vi "手动界面.vi"(8 "错误输入（无错误）":errorcluster, 10 "界面切换队列":refnum<queue>, 11 "VISA资源名称输入":refnum<visa-resource-name>) -> (0 "错误输出":errorcluster, 3 "VISA资源名称输出":refnum<visa-resource-name>)   [LabVIEW 2018]
panel:
  out "毫秒计时值":u32
  in  "枚举":T1(ring)
  out "选项卡控件":enum32{"选项卡 1", "选项卡 2"}(tab)
  out "写R2E+读Y1C+2号吸嘴真空":bool
  out "写R2C+读Y1B+1号吸嘴真空":bool
  out "写R2A+读Y13+真空泵":bool
  out "写R81+读R81+切换+快速":bool
  out "写R2D+读Y16+2号吸嘴吹气":bool
  out "写R2B+读Y14+1号吸嘴吹气":bool
  out "烧录座手动界面":bool
  out "写R1F+读R5F+R2轴旋转定位":bool
  out "写R1C+读R5C+R1轴旋转定位":bool
  in  "DT63+枚举":enum16{"90度", "180度", "270度"}(ring)
  in  "DT62+枚举":enum16{"90度", "180度", "270度"}(ring)
  out "写R25+读YC+卷带信号":bool
  out "写R26+读YD+换盘信号":bool
  out "写R19+读R59+Z2轴+":bool
  out "写R16+读R56+Z轴+":bool
  out "写R168+读R168+切换+手柄Z1轴":bool
  out "写R1A+读R5A+Z2轴-":bool
  out "写R17+读R57+Z1轴-":bool
  out "写R20+读Y19+2#飞达信号":bool
  out "写R2F+读Y18+1#飞达信号":bool
  out "写R1B+读R5B+Z2轴回原点":bool
  out "写R18+读R58+Z轴回原点":bool
  out "手动2界面":bool
  out "写R80+读R80+报警清除":bool
  out "写R8+读R9+机器复位":bool
  out "写R4+读R4+手动停止":bool
  out "写R0+读R1+手动启动":bool
  out "写R11+读R51+X轴-":bool
  out "写R10+读R50+X轴+":bool
  out "写R13+读R53+Y轴+":bool
  out "写R14+读R54+Y轴-":bool
  out "写R15+读R55+Y轴回原点":bool
  out "写R12+读R52+X轴回原点":bool
  out "DDT90356":dbl
  out "DDT90348":dbl
  out "自动界面":bool
  out "手动界面":bool
  out "参数界面":bool
  out "IO界面":bool
  out "产品界面":bool
  out "字符串":string
  out "DDT90352":dbl
  out "DDT90360":dbl
  out "DT1184":T2(ring)
  out "通讯周期":dbl
  # "X"
  # "Z1"
  # "Z2"
  # "Y"
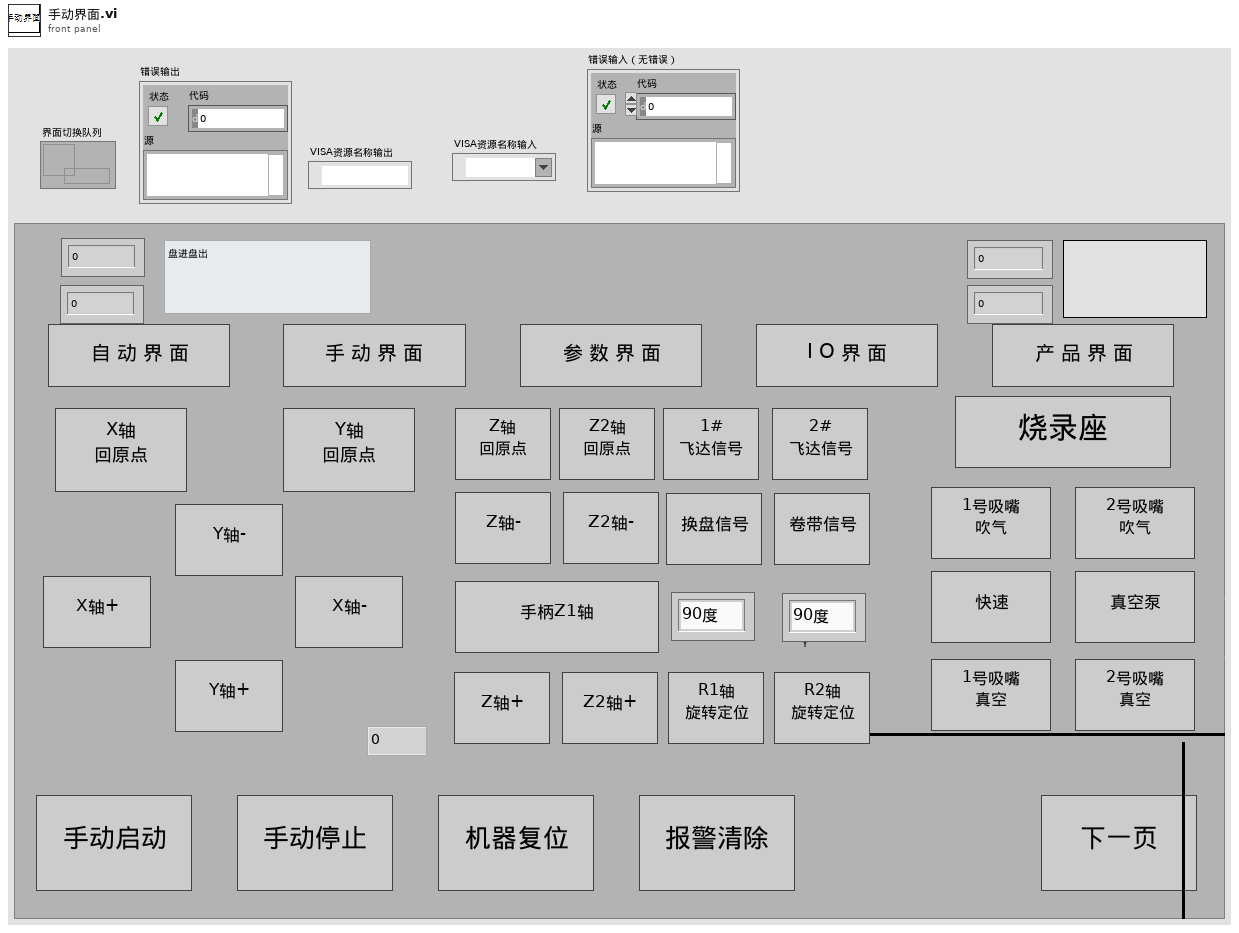
[diagram p1: front panel]
types:
  T1 = enum16{"读初始化", "读DT62+8", "读R168+8", "读R80+8", "读YC+8", "读Y1B+8", "读Y13+8", "读R9+8", "读R1+8", "读R50+8", "读R58+8", "读DDT90356", "读DT1184", "读DDT90348", ""}
  T2 = enum16{"盘进盘出", "卷进卷出", "盘进卷出", "管进盘出", "管进卷出", "卷进盘出", ""}
  T3 = enum8{"Enabled", "Disabled", "Disabled and Grayed Out"}
  T4 = typedef "数据簇.ctl" = cluster{"字符串":string, "数值":i32, "布尔":bool}
  T5 = typedef "lveventtype.ctl" = enum32{"Null", "Timeout", "Annotation Menu Selection", "Annotation Menu Selection?", "App Instance Close", "App Instance Close?", "Autoscale Range Change", "Bookmark Info Change", "Cell Edit", "Cell Edit?", "Cursor Grab", "Cursor Grab?", "Cursor Menu Selection", "Cursor Menu Selection?", "Cursor Move", "Cursor Release", "Data Change", "Direction Change", "Display State Change", "Drag Ended", "Drag Enter", "Drag Leave", "Drag Over", "Drag Source Update", "Drag Starting", "Drag Starting?", "Drop", "Exec State Change", "Key Down", "Key Down?", "Key Repeat", "Key Repeat?", "Key Up", "Listbox Double Click", "Menu Activation?", "Menu Selection (App)", "Menu Selection? (App)", "Menu Selection (User)", "Mouse Down", "Mouse Down?", "Mouse Enter", "Mouse Leave", "Mouse Move", "Mouse Up", "Mouse Wheel", "NI Security User Change (App)", "Pane Size", "Panel Close", "Panel Close?", "Panel Resize", "Plot Attribute Change", "Scale Range Change", "Shortcut Menu Activation?", "Shortcut Menu Selection (App)", "Shortcut Menu Selection? (App)", "Shortcut Menu Selection (User)", "Tree Double Click", "Tree Drag", "Tree Drag?", "Tree Drop", "Tree Drop?", "Tree Item Close", "Tree Item Close?", "Tree Item Open", "Tree Item Open?", "User Event", "Value Change"}
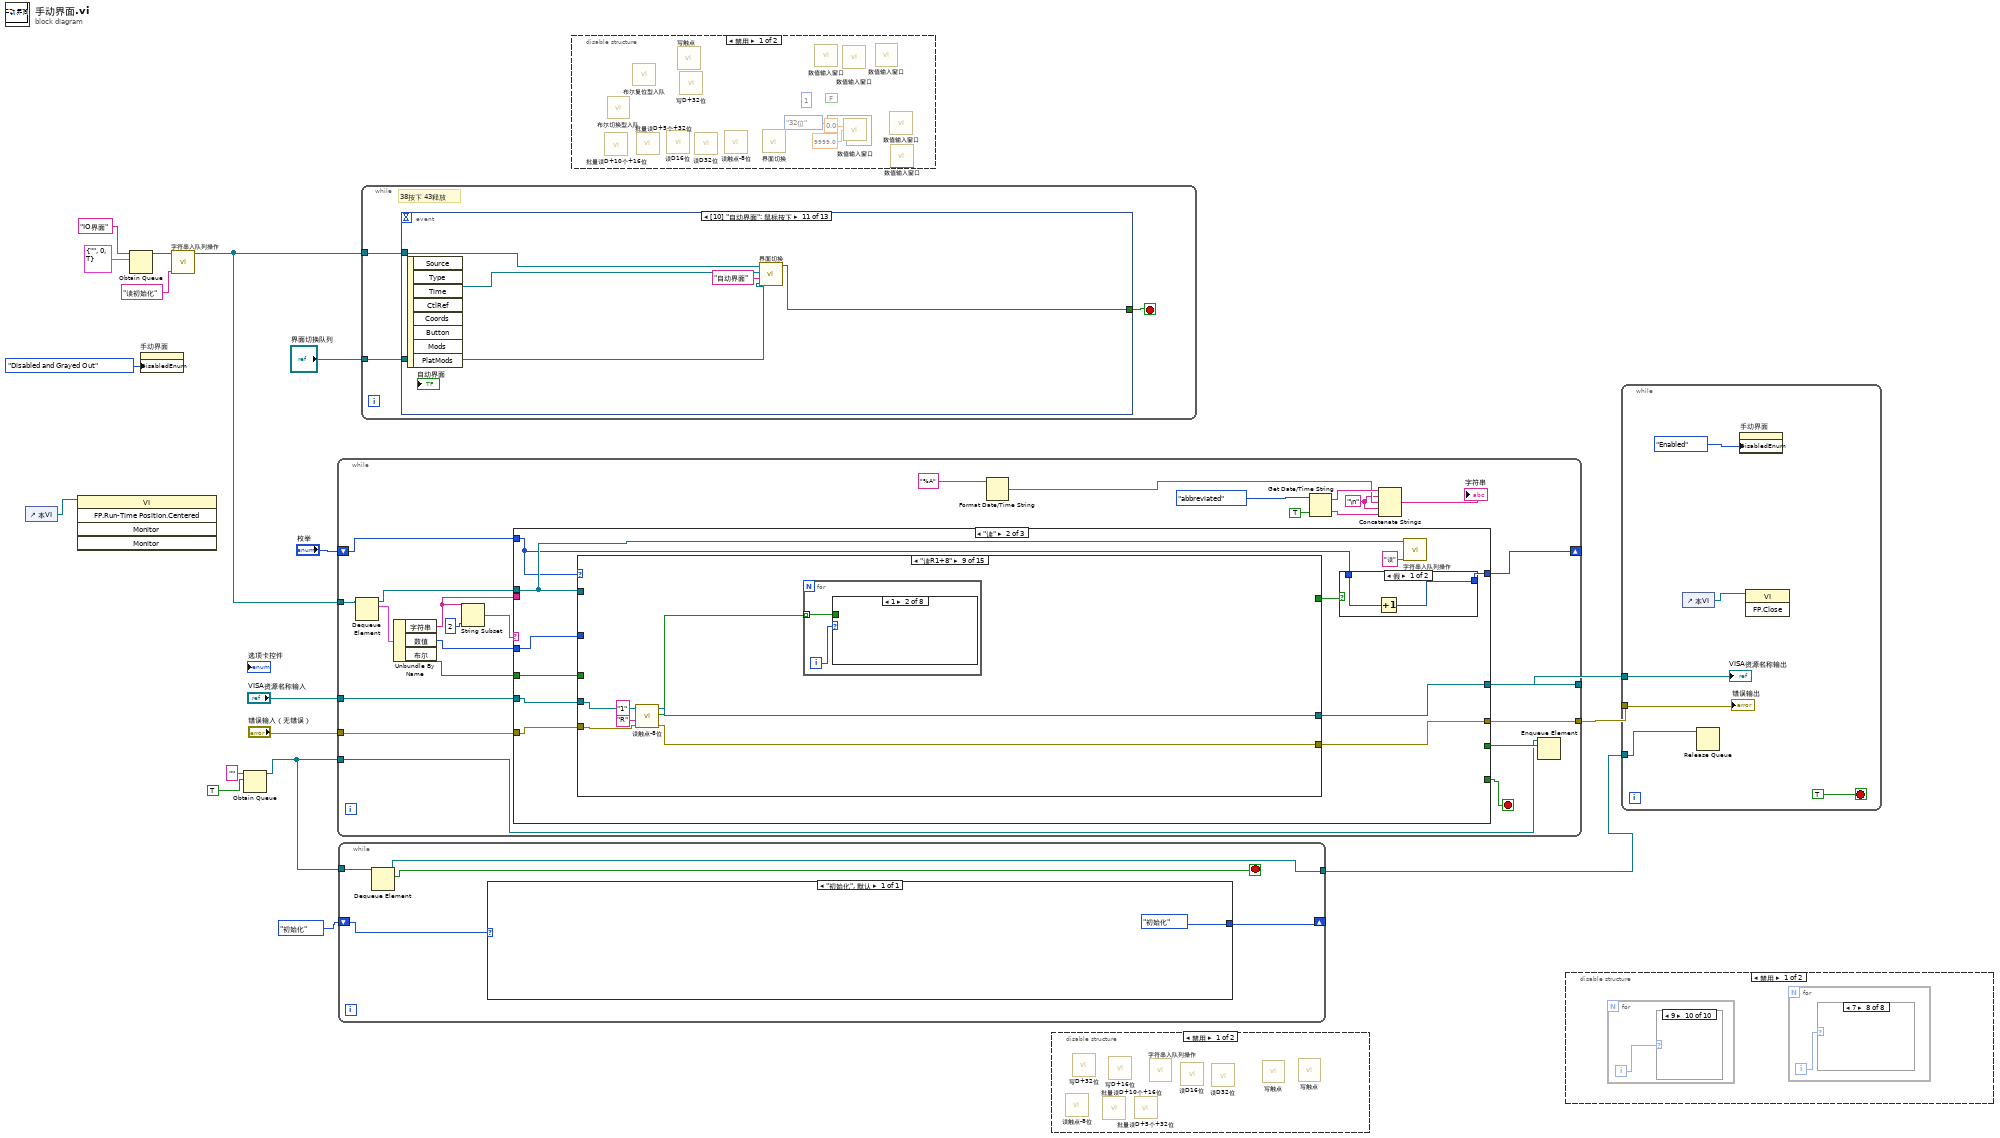
[diagram p0: block diagram]
diagram:
  n1 = control-ref of="本VI"() -> (w2:refnum<vi>)
  n2 = invoke class="VI" method="FP.Run-Time Position.Centered"(reference=w2) -> ()  [unwired: 4 in, 5 out]
  n3 = Obtain Queue(name (unnamed)="IO界面" ("名称（未命名）"), element data type=T4 {"字符串"="", "数值"=0, "布尔"=TRUE}) -> (queue out=w11:refnum<queue>)  [unwired: 3 in, 2 out]
  n4 = property on="手动界面" class="Bool"("DisabledEnum"=T3."Disabled and Grayed Out" ("禁用")) -> ()  [unwired: 2 in, 2 out]
  n5 = call "字符串入队列操作.vi"("字符消息入队列"="读初始化", "界面切换队列"=w11) -> ("队列输出"=w3:refnum<queue>)  [unwired: 9 in]
  n6 = Obtain Queue(name (unnamed)="" ("名称（未命名）"), element data type=TRUE) -> (queue out=w6:refnum<queue>)  [unwired: 3 in, 2 out]
  n7 = while {
    tunnel: w3 -> [w39]
    tunnel: "VISA资源名称输入" -> [w32]
    tunnel: "错误输入（无错误）" -> [w31]
    tunnel: [w30] -> w13
    tunnel: [w29] -> w12
    shift-right: [w26] -> _
    shift-left: "枚举" -> [w27]
    tunnel: w6 -> [w19]
    stop <- w21 stop-if-true
    w23 = "\n"
    n8 = Dequeue Element(queue=w39) -> (queue out=w36:refnum<queue>, element=w38:T4)  [unwired: 2 in, 2 out]
    n9 = Unbundle By Name(w38) -> ("字符串"=w33:string, "数值"=w35:i32, "布尔"=w34:bool)
    n10 = String Subset(string=w33, length (rest)=2 ("长度（剩余）")) -> (substring=w37:string)  [unwired: 1 in]
    n11 = case shown="\"读\"" w37 {
      selector: w37 -> [w46 _ _]
      tunnel: w36 -> [_ w54 w243]
      tunnel: w35 -> [_ w61 w242]
      tunnel: w34 -> [_ w60 w241]
      tunnel: w33 -> [_ _ w235]
      tunnel: w32 -> [w45 w59 w240]
      tunnel: w31 -> [w44 w58 w239]
      tunnel: [w45 w57 w237] -> w30
      tunnel: [w44 w56 w236] -> w29
      tunnel: [_ _ w238] -> w21
      tunnel: w27 -> [_ w52 _]
      tunnel: [_ w51 _] -> w26
      tunnel: [_ _ w233] -> w20
      frame "", Default {
        n12 = Concatenate Strings("无对应消息分支**" ("消息"), w46, "**" ("字符串"), "读写状态机" ("字符串")) -> (w48:string)
        n13 = One Button Dialog(message=w48) -> ()  [unwired: 1 in, 1 out]
      }
      frame "读" {
        n14 = case shown="\"读R1+8\"" w52 {
          tunnel: w54 -> [_ _ _ _ _ _ _ _ _ _ _ _ _ _ _]
          tunnel: w61 -> [_ _ _ _ _ _ _ _ _ _ _ _ _ _ _]
          tunnel: w59 -> [w66 w72 w83 w93 w104 w115 w126 w140 w150 w161 w178 w198 w207 w220 w232]
          tunnel: w58 -> [w65 w71 w82 w92 w103 w114 w125 w139 w149 w160 w177 w197 w206 w219 w231]
          tunnel: [w66 w69 w79 w91 w100 w113 w124 w136 w146 w157 w176 w196 w205 w218 w232] -> w57
          tunnel: [w65 w68 w78 w90 w99 w112 w123 w135 w145 w156 w175 w195 w204 w217 w231] -> w56
          tunnel: w60 -> [_ _ _ _ _ _ _ _ _ _ _ _ _ _ _]
          tunnel: [_ _ _ _ _ _ _ _ _ _ _ _ _ _ TRUE] -> w53
          frame "读初始化" {
            n15 = Tick Count (ms)() -> (millisecond timer value=→"毫秒计时值":u32)
          }
          frame "读DT62+8" {
            n16 = call "批量读D+10个+16位.vi"("error out"=w71, "读取D地址"=62, "VISA resource name out"=w72) -> ("error IO"=w68:errorcluster, "数组"=w67:i32[], "VISA resource name out 2"=w69:refnum<visa-resource-name>)  [unwired: 5 in, 1 out]
            n17 = for {
              tunnel: w67 -> [w73] mode=indexing
              i -> [w74]
              n18 = case shown="1" w74 {
                tunnel: w73 -> [w75 w76 _ _ _ _ _ _ _ _]
                frame 0, Default {
                  n19 = local write "DT62+枚举"(w75) -> ()
                }
                frame 1 {
                  n20 = local write "DT63+枚举"(w76) -> ()
                }
                frame 2 {
                }
                frame 3 {
                }
                frame 4 {
                }
                frame 5 {
                }
                frame 6 {
                }
                frame 7 {
                }
                frame 8 {
                }
                frame 9 {
                }
              }
            }
          }
          frame "读R168+8" {
            n21 = call "读触点-8位.vi"("error out"=w82, "触点类型"="R", "读取起始地址"="168", "VISA resource name out"=w83) -> ("error IO"=w78:errorcluster, "读取布尔数组"=w77:bool[], "VISA resource name out 2"=w79:refnum<visa-resource-name>)  [unwired: 4 in, 1 out]
            n22 = for {
              tunnel: w77 -> [w84] mode=indexing
              i -> [w85]
              n23 = case shown="0, 默认" w85 {
                tunnel: w84 -> [w86 _ _ _ _ _ _ _]
                frame 0, Default {
                  "写R168+读R168+切换+手柄Z1轴" <- w86
                }
                frame 1 {
                }
                frame 2 {
                }
                frame 3 {
                }
                frame 4 {
                }
                frame 5 {
                }
                frame 6 {
                }
                frame 7 {
                }
              }
            }
          }
          frame "读R80+8" {
            n24 = call "读触点-8位.vi"("error out"=w92, "触点类型"="R", "读取起始地址"="80", "VISA resource name out"=w93) -> ("error IO"=w90:errorcluster, "读取布尔数组"=w87:bool[], "VISA resource name out 2"=w91:refnum<visa-resource-name>)  [unwired: 4 in, 1 out]
            n25 = for {
              tunnel: w87 -> [w94] mode=indexing
              i -> [w95]
              n26 = case shown="0, 默认" w95 {
                tunnel: w94 -> [w96 w97 _ _ _ _ _ _]
                frame 0, Default {
                  "写R80+读R80+报警清除" <- w96
                }
                frame 1 {
                  "写R81+读R81+切换+快速" <- w97
                }
                frame 2 {
                }
                frame 3 {
                }
                frame 4 {
                }
                frame 5 {
                }
                frame 6 {
                }
                frame 7 {
                }
              }
            }
          }
          frame "读YC+8" {
            n27 = call "读触点-8位.vi"("error out"=w103, "触点类型"="Y", "读取起始地址"="C", "VISA resource name out"=w104) -> ("error IO"=w99:errorcluster, "读取布尔数组"=w98:bool[], "VISA resource name out 2"=w100:refnum<visa-resource-name>)  [unwired: 4 in, 1 out]
            n28 = for {
              tunnel: w98 -> [w105] mode=indexing
              i -> [w106]
              n29 = case shown="1" w106 {
                tunnel: w105 -> [w107 w108 _ _ _ _ _ _]
                frame 0, Default {
                  "写R25+读YC+卷带信号" <- w107
                }
                frame 1 {
                  "写R26+读YD+换盘信号" <- w108
                }
                frame 2 {
                }
                frame 3 {
                }
                frame 4 {
                }
                frame 5 {
                }
                frame 6 {
                }
                frame 7 {
                }
              }
            }
          }
          frame "读Y1B+8" {
            n30 = call "读触点-8位.vi"("error out"=w114, "触点类型"="Y", "读取起始地址"="1C", "VISA resource name out"=w115) -> ("error IO"=w112:errorcluster, "读取布尔数组"=w111:bool[], "VISA resource name out 2"=w113:refnum<visa-resource-name>)  [unwired: 4 in, 1 out]
            n31 = for {
              tunnel: w111 -> [w116] mode=indexing
              i -> [w117]
              n32 = case shown="1" w117 {
                tunnel: w116 -> [w118 w119 _ _ _ _ _ _]
                frame 0, Default {
                  "写R2C+读Y1B+1号吸嘴真空" <- w118
                }
                frame 1 {
                  "写R2E+读Y1C+2号吸嘴真空" <- w119
                }
                frame 2 {
                }
                frame 3 {
                }
                frame 4 {
                }
                frame 5 {
                }
                frame 6 {
                }
                frame 7 {
                }
              }
            }
          }
          frame "读Y13+8" {
            n33 = call "读触点-8位.vi"("error out"=w125, "触点类型"="Y", "读取起始地址"="13", "VISA resource name out"=w126) -> ("error IO"=w123:errorcluster, "读取布尔数组"=w122:bool[], "VISA resource name out 2"=w124:refnum<visa-resource-name>)  [unwired: 4 in, 1 out]
            n34 = for {
              tunnel: w122 -> [w127] mode=indexing
              i -> [w128]
              n35 = case shown="6" w128 {
                tunnel: w127 -> [w129 w130 _ w131 _ w132 w133 _]
                frame 0, Default {
                  "写R2A+读Y13+真空泵" <- w129
                }
                frame 1 {
                  "写R2B+读Y14+1号吸嘴吹气" <- w130
                }
                frame 2 {
                }
                frame 3 {
                  "写R2D+读Y16+2号吸嘴吹气" <- w131
                }
                frame 4 {
                }
                frame 5 {
                  "写R2F+读Y18+1#飞达信号" <- w132
                }
                frame 6 {
                  "写R20+读Y19+2#飞达信号" <- w133
                }
                frame 7 {
                }
              }
            }
          }
          frame "读R9+8" {
            n36 = call "读触点-8位.vi"("error out"=w139, "触点类型"="R", "读取起始地址"="9", "VISA resource name out"=w140) -> ("error IO"=w135:errorcluster, "读取布尔数组"=w134:bool[], "VISA resource name out 2"=w136:refnum<visa-resource-name>)  [unwired: 4 in, 1 out]
            n37 = for {
              tunnel: w134 -> [w141] mode=indexing
              i -> [w142]
              n38 = case shown="0, 默认" w142 {
                tunnel: w141 -> [w143 _ _ _ _ _ _ _]
                frame 0, Default {
                  "写R8+读R9+机器复位" <- w143
                }
                frame 1 {
                }
                frame 2 {
                }
                frame 3 {
                }
                frame 4 {
                }
                frame 5 {
                }
                frame 6 {
                }
                frame 7 {
                }
              }
            }
          }
          frame "读R1+8" {
            n39 = call "读触点-8位.vi"("error out"=w149, "触点类型"="R", "读取起始地址"="1", "VISA resource name out"=w150) -> ("error IO"=w145:errorcluster, "读取布尔数组"=w144:bool[], "VISA resource name out 2"=w146:refnum<visa-resource-name>)  [unwired: 4 in, 1 out]
            n40 = for {
              tunnel: w144 -> [w151] mode=indexing
              i -> [w152]
              n41 = case shown="1" w152 {
                tunnel: w151 -> [w153 _ _ w154 _ _ _ _]
                frame 0, Default {
                  "写R0+读R1+手动启动" <- w153
                }
                frame 1 {
                }
                frame 2 {
                }
                frame 3 {
                  "写R4+读R4+手动停止" <- w154
                }
                frame 4 {
                }
                frame 5 {
                }
                frame 6 {
                }
                frame 7 {
                }
              }
            }
          }
          frame "读R50+8" {
            n42 = call "读触点-8位.vi"("error out"=w160, "触点类型"="R", "读取起始地址"="50", "VISA resource name out"=w161) -> ("error IO"=w156:errorcluster, "读取布尔数组"=w155:bool[], "VISA resource name out 2"=w157:refnum<visa-resource-name>)  [unwired: 4 in, 1 out]
            n43 = for {
              tunnel: w155 -> [w162] mode=indexing
              i -> [w163]
              n44 = case shown="7" w163 {
                tunnel: w162 -> [w164 w165 w166 w167 w168 w169 w170 w171]
                frame 0, Default {
                  "写R10+读R50+X轴+" <- w164
                }
                frame 1 {
                  "写R11+读R51+X轴-" <- w165
                }
                frame 2 {
                  "写R12+读R52+X轴回原点" <- w166
                }
                frame 3 {
                  "写R13+读R53+Y轴+" <- w167
                }
                frame 4 {
                  "写R14+读R54+Y轴-" <- w168
                }
                frame 5 {
                  "写R15+读R55+Y轴回原点" <- w169
                }
                frame 6 {
                  "写R16+读R56+Z轴+" <- w170
                }
                frame 7 {
                  "写R17+读R57+Z1轴-" <- w171
                }
              }
            }
          }
          frame "读R58+8" {
            n45 = call "读触点-8位.vi"("error out"=w177, "触点类型"="R", "读取起始地址"="58", "VISA resource name out"=w178) -> ("error IO"=w175:errorcluster, "读取布尔数组"=w172:bool[], "VISA resource name out 2"=w176:refnum<visa-resource-name>)  [unwired: 4 in, 1 out]
            n46 = for {
              tunnel: w172 -> [w179] mode=indexing
              i -> [w180]
              n47 = case shown="7" w180 {
                tunnel: w179 -> [w181 w182 w183 w184 w185 _ _ w186]
                frame 0, Default {
                  "写R18+读R58+Z轴回原点" <- w181
                }
                frame 1 {
                  "写R19+读R59+Z2轴+" <- w182
                }
                frame 2 {
                  "写R1A+读R5A+Z2轴-" <- w183
                }
                frame 3 {
                  "写R1B+读R5B+Z2轴回原点" <- w184
                }
                frame 4 {
                  "写R1C+读R5C+R1轴旋转定位" <- w185
                }
                frame 5 {
                }
                frame 6 {
                }
                frame 7 {
                  "写R1F+读R5F+R2轴旋转定位" <- w186
                }
              }
            }
          }
          frame "读DDT90356" {
            n48 = call "批量读D+5个+32位.vi"("error out"=w197, "读取D地址"=90356, "VISA resource name out"=w198) -> ("error IO"=w195:errorcluster, "数组"=w201:i32[], "VISA resource name out 2"=w196:refnum<visa-resource-name>)  [unwired: 5 in, 1 out]
            n49 = Index Array(array=w201, index #1=0 ("索引"), index #2=2 ("索引")) -> (element #1=w194:i32, element #2=w193:i32)
            n50 = To Double Precision Float(number=w194) -> (double precision float=w192:dbl)
            n51 = To Double Precision Float(number=w193) -> (double precision float=w189:dbl)
            n52 = Divide(x=w192, y=100.0) -> (x/y=→"DDT90356":dbl)
            n53 = Divide(x=w189, y=100.0) -> (x/y=→"DDT90360":dbl)
          }
          frame "读DT1184" {
            n54 = call "读D16位.vi"("error out"=w206, "读取D地址"=1184, "VISA resource name out"=w207) -> ("error IO"=w204:errorcluster, "数值"=→"DT1184":u32, "VISA resource name out 2"=w205:refnum<visa-resource-name>)  [unwired: 5 in, 1 out]
          }
          frame "读DDT90348" {
            n55 = call "批量读D+5个+32位.vi"("error out"=w219, "读取D地址"=90348, "VISA resource name out"=w220) -> ("error IO"=w217:errorcluster, "数组"=w224:i32[], "VISA resource name out 2"=w218:refnum<visa-resource-name>)  [unwired: 5 in, 1 out]
            n56 = Index Array(array=w224, index #1=0 ("索引"), index #2=2 ("索引")) -> (element #1=w216:i32, element #2=w215:i32)
            n57 = To Double Precision Float(number=w215) -> (double precision float=w210:dbl)
            n58 = To Double Precision Float(number=w216) -> (double precision float=w214:dbl)
            n59 = Divide(x=w210, y=100.0) -> (x/y=→"DDT90352":dbl)
            n60 = Divide(x=w214, y=100.0) -> (x/y=→"DDT90348":dbl)
          }
          frame "" {
            n61 = local read "毫秒计时值"() -> (w228:u32)
            n62 = Tick Count (ms)() -> (millisecond timer value=w229:u32)
            n63 = Subtract(x=w229, y=w228) -> (x-y=w227:u32)
            n64 = Divide(x=w227, y=u32 1000) -> (x/y=→"通讯周期":dbl)
          }
        }
        n65 = case shown="假" w53 {
          tunnel: w52 -> [w63 _]
          tunnel: [w62 _] -> w51
          frame False {
            n66 = Increment(x=w63) -> (x+1=w62:T1)
          }
          frame True {
          }
        }
        n67 = call "字符串入队列操作.vi"("字符消息入队列"="读", "界面切换队列"=w54) -> ()  [unwired: 9 in, 1 out]
      }
      frame "写" {
        n68 = call "状态匹配.vi"("输入状态"=w235) -> ("输出状态"=w234:string)  [unwired: 10 in]
        n69 = case shown="\"写DT\"" w234 {
          selector: w234 -> [w246 _ _ _ _]
          tunnel: w243 -> [_ _ _ _ w286]
          tunnel: w242 -> [_ w252 w269 _ _]
          tunnel: w241 -> [_ _ _ w280 _]
          tunnel: w240 -> [w245 w262 w273 w285 w291]
          tunnel: w239 -> [w244 w261 w272 w284 w290]
          tunnel: [_ _ _ _ w289] -> w238
          tunnel: [w245 w260 w271 w283 w291] -> w237
          tunnel: [w244 w259 w270 w282 w290] -> w236
          tunnel: w235 -> [_ w251 w263 w274 _]
          tunnel: [_ _ _ _ w289] -> w233
          frame "", Default {
            n70 = Concatenate Strings("无对应消息分支**" ("消息"), w246, "**" ("字符串"), "写状态机" ("字符串")) -> (w250:string)
            n71 = One Button Dialog(message=w250) -> ()  [unwired: 1 in, 1 out]
          }
          frame "写DT" {
            n72 = String Length(string=w251) -> (length=w257:i32)
            n73 = Subtract(x=w257, y=4) -> (x-y=w255:i32)
            n74 = String Subset(string=w251, offset (0)=4 ("偏移量(0)"), length (rest)=w255) -> (substring=w254:string)
            n75 = Decimal String To Number(string=w254) -> (number=w253:i32)  [unwired: 2 in, 1 out]
            n76 = call "写D+16位.vi"("error out"=w261, "输入数值"=w252, "输入地址D"=w253, "VISA resource name out"=w262) -> ("error out 2"=w259:errorcluster, "VISA resource name out 2"=w260:refnum<visa-resource-name>)  [unwired: 3 in, 3 out]
          }
          frame "写DDT" {
            n77 = String Length(string=w263) -> (length=w267:i32)
            n78 = Subtract(x=w267, y=5) -> ()  [unwired: 1 out]
            n79 = String Subset(string=w263, offset (0)=5 ("偏移量(0)")) -> (substring=w264:string)  [unwired: 1 in]
            n80 = Decimal String To Number(string=w264) -> (number=w265:i32)  [unwired: 2 in, 1 out]
            n81 = call "写D+32位.vi"("error out"=w272, "输入数值"=w269, "输入地址D"=w265, "VISA resource name out"=w273) -> ("error out 2"=w270:errorcluster, "VISA resource name out 2"=w271:refnum<visa-resource-name>)  [unwired: 4 in, 2 out]
          }
          frame "写R" {
            n82 = String Length(string=w274) -> (length=w278:i32)
            n83 = Subtract(x=w278, y=3) -> (x-y=w276:i32)
            n84 = String Subset(string=w274, offset (0)=3 ("偏移量(0)"), length (rest)=w276) -> (substring=w275:string)
            n85 = call "写触点.vi"("布尔"=w280, "error out"=w284, "触点类型"="R", "写入起始地址"=w275, "VISA resource name out"=w285) -> ("error IO"=w282:errorcluster, "VISA resource name out 2"=w283:refnum<visa-resource-name>)  [unwired: 4 in, 1 out]
          }
          frame "写退出" {
            w289 = TRUE
            n86 = Flush Queue(queue=w286) -> (queue out=w287:refnum<queue>, error out=w288:errorcluster)  [unwired: 1 in, 1 out]
            n87 = Release Queue(queue=w287, error in (no error)=w288) -> ()  [unwired: 1 in, 3 out]
          }
        }
      }
    }
    n88 = Format Date/Time String(time format string (%c)="%A" ("时间格式字符串(%c)")) -> (date/time string=w24:string)  [unwired: 2 in]
    n89 = Get Date/Time String(date format (0)=enum16{"short", "long", "abbreviated"}."abbreviated" ("日期格式(0)"), want seconds? (F)=TRUE ("需要秒？(F)")) -> (date string=w41:string, time string=w22:string)  [unwired: 1 in]
    n90 = Concatenate Strings(w41, w23, w24, w23, w22) -> (→"字符串":string)
    n91 = Enqueue Element(queue=w19, element=w20) -> ()  [unwired: 2 in, 3 out]
  }
  n92 = while {
    shift-right: [w295] -> _
    shift-left: enum16{"初始化"}."初始化" -> [w296]
    tunnel: w6 -> [w294]
    tunnel: [w292] -> w5
    stop <- w293 stop-if-true
    n93 = Dequeue Element(queue=w294) -> (queue out=w292:refnum<queue>, element=w293:bool)  [unwired: 2 in, 2 out]
    n94 = case shown="\"初始化\", 默认" w296 {
      tunnel: [enum16{"初始化"}."初始化"] -> w295
      frame "初始化", Default {
      }
    }
  }
  n95 = while {
    tunnel: w3 -> [w299]
    tunnel: "界面切换队列" -> [w298]
    stop <- w300 stop-if-true
    # "38按下 43释放"
    n96 = event shown="[10] \"自动界面\": 鼠标按下" {
      selector: _ -> [_ _ _ _ _ _ _ _ _ _ _ _ _]
      dyn-events: _ -> [_ _ _ _ _ _ _ _ _ _ _ _ _]
      timeout: _ -> [_ _ _ _ _ _ _ _ _ _ _ _ _]
      tunnel: [w304 _ _ w316 _ _ w331 w340 w345 w346 w355 _ w358] -> w300
      tunnel: w299 -> [w305 w308 w315 w320 w327 w330 w335 w339 w344 w350 w354 _ w357]
      tunnel: w298 -> [w303 _ _ w319 _ _ w334 w338 w343 w349 w353 _ w356]
      event "IO界面": Mouse Down {
        n97 = event-data() -> ("CtlRef"=w302:refnum<vi>)  [unwired: 1 in, 7 out]
        n98 = call "界面切换.vi"("界面切换队列输入"=w303, "切换界面名称输入"="IO界面", "Bool引用句柄"=w302, "状态转移输入"=w305) -> ("布尔"=w304:bool)  [unwired: 7 in]
      }
      event "DT62+枚举": Value Change {
        n99 = event-data() -> ("NewVal"=w306:enum16{"90度", "180度", "270度"})  [unwired: 1 in, 5 out]
        n100 = call "字符串入队列操作.vi"("字符消息入队列"="写DT62", "数值"=w306, "界面切换队列"=w308) -> ()  [unwired: 8 in, 1 out]
      }
      event "写R12+读R52+X轴回原点", "写R15+读R55+Y轴回原点", "写R14+读R54+Y轴-", "写R13+读R53+Y轴+", "写R10+读R50+X轴+", "写R11+读R51+X轴-", "写R0+读R1+手动启动", "写R4+读R4+手动停止", "写R8+读R9+机器复位", "写R80+读R80+报警清除", "写R18+读R58+Z轴回原点", "写R1B+读R5B+Z2轴回原点", "写R2F+读Y18+1#飞达信号", "写R20+读Y19+2#飞达信号", "写R17+读R57+Z1轴-", "写R1A+读R5A+Z2轴-", "写R16+读R56+Z轴+", "写R19+读R59+Z2轴+", "写R26+读YD+换盘信号", "写R25+读YC+卷带信号", "写R1C+读R5C+R1轴旋转定位", "写R1F+读R5F+R2轴旋转定位", "写R2B+读Y14+1号吸嘴吹气", "写R2D+读Y16+2号吸嘴吹气", "写R2A+读Y13+真空泵", "写R2C+读Y1B+1号吸嘴真空", "写R2E+读Y1C+2号吸嘴真空": Mouse Down; "写R12+读R52+X轴回原点", "写R15+读R55+Y轴回原点", "写R14+读R54+Y轴-", "写R13+读R53+Y轴+", "写R10+读R50+X轴+", "写R11+读R51+X轴-", "写R0+读R1+手动启动", "写R8+读R9+机器复位", "写R80+读R80+报警清除", "写R18+读R58+Z轴回原点", "写R1B+读R5B+Z2轴回原点", "写R2F+读Y18+1#飞达信号", "写R20+读Y19+2#飞达信号", "写R17+读R57+Z1轴-", "写R1A+读R5A+Z2轴-", "写R16+读R56+Z轴+", "写R19+读R59+Z2轴+", "写R26+读YD+换盘信号", "写R25+读YC+卷带信号", "写R1C+读R5C+R1轴旋转定位", "写R2B+读Y14+1号吸嘴吹气", "写R2D+读Y16+2号吸嘴吹气", "写R2A+读Y13+真空泵", "写R2C+读Y1B+1号吸嘴真空", "写R2E+读Y1C+2号吸嘴真空", "写R4+读R4+手动停止": Mouse Up {
        n101 = event-data() -> ("Type"=w314:T5, "CtlRef"=w313:refnum<vi>)  [unwired: 1 in, 6 out]
        n102 = property class="Bool"(reference=w313) -> (reference out=w310:refnum<vi>, "Label.Text"=w312:string)  [unwired: 1 in, 1 out]
        n103 = Match Pattern(string=w312, regular expression="+" ("正则表达式")) -> (before substring=w309:string)  [unwired: 1 in, 3 out]
        n104 = call "布尔复位型入队.vi"("队列输入"=w315, "数值"=w314, "控件引用"=w310, "字符消息入队列"=w309) -> ()  [unwired: 2 in, 3 out]
      }
      event "烧录座手动界面": Mouse Down {
        n105 = event-data() -> ("CtlRef"=w318:refnum<vi>)  [unwired: 1 in, 7 out]
        n106 = call "界面切换.vi"("界面切换队列输入"=w319, "切换界面名称输入"="烧录座手动界面", "Bool引用句柄"=w318, "状态转移输入"=w320) -> ("布尔"=w316:bool)  [unwired: 7 in]
      }
      event "写R81+读R81+切换+快速", "写R168+读R168+切换+手柄Z1轴": Mouse Down {
        n107 = event-data() -> ("CtlRef"=w323:refnum<vi>)  [unwired: 1 in, 7 out]
        n108 = property class="Bool"(reference=w323) -> (reference out=w322:refnum<vi>, "Label.Text"=w325:string)  [unwired: 1 in, 1 out]
        n109 = Match Pattern(string=w325, regular expression="+" ("正则表达式")) -> (before substring=w321:string)  [unwired: 1 in, 3 out]
        n110 = call "布尔切换型入队.vi"("字符串"=w321, "true启用入队"=TRUE, "控件引用"=w322, "消息入队列"=w327) -> ()  [unwired: 8 in]
      }
      event "DT63+枚举": Value Change {
        n111 = event-data() -> ("NewVal"=w328:enum16{"90度", "180度", "270度"})  [unwired: 1 in, 5 out]
        n112 = call "字符串入队列操作.vi"("字符消息入队列"="写DT63", "数值"=w328, "界面切换队列"=w330) -> ()  [unwired: 8 in, 1 out]
      }
      event "手动2界面": Mouse Down {
        n113 = event-data() -> ("CtlRef"=w333:refnum<vi>)  [unwired: 1 in, 7 out]
        n114 = call "界面切换.vi"("界面切换队列输入"=w334, "切换界面名称输入"="手动2界面", "Bool引用句柄"=w333, "状态转移输入"=w335) -> ("布尔"=w331:bool)  [unwired: 7 in]
      }
      event "参数界面": Mouse Down {
        n115 = event-data() -> ("CtlRef"=w337:refnum<vi>)  [unwired: 1 in, 7 out]
        n116 = call "界面切换.vi"("界面切换队列输入"=w338, "切换界面名称输入"="参数界面", "Bool引用句柄"=w337, "状态转移输入"=w339) -> ("布尔"=w340:bool)  [unwired: 7 in]
      }
      event "产品界面": Mouse Down {
        n117 = event-data() -> ("CtlRef"=w342:refnum<vi>)  [unwired: 1 in, 7 out]
        n118 = call "界面切换.vi"("界面切换队列输入"=w343, "切换界面名称输入"="产品界面", "Bool引用句柄"=w342, "状态转移输入"=w344) -> ("布尔"=w345:bool)  [unwired: 7 in]
      }
      event "手动界面": Mouse Down {
        n119 = event-data() -> ("CtlRef"=w348:refnum<vi>)  [unwired: 1 in, 7 out]
        n120 = call "界面切换.vi"("界面切换队列输入"=w349, "切换界面名称输入"="手动界面", "Bool引用句柄"=w348, "状态转移输入"=w350) -> ("布尔"=w346:bool)  [unwired: 7 in]
      }
      event "自动界面": Mouse Down {
        n121 = event-data() -> ("CtlRef"=w352:refnum<vi>)  [unwired: 1 in, 7 out]
        n122 = call "界面切换.vi"("界面切换队列输入"=w353, "切换界面名称输入"="自动界面", "Bool引用句柄"=w352, "状态转移输入"=w354) -> ("布尔"=w355:bool)  [unwired: 7 in]
      }
      event Timeout {
        n123 = event-data() -> ()  [unwired: 1 in, 3 out]
      }
      event Panel Close? {
        n124 = event-data() -> ()  [unwired: 1 in, 4 out]
        n125 = Two Button Dialog(message="确定退出程序？" ("消息")) -> (T button?=w359:bool)  [unwired: 2 in]
        n126 = case shown="真" w359 {
          tunnel: [_ TRUE] -> w358
          tunnel: w357 -> [_ w364]
          tunnel: w356 -> [_ w363]
          frame False {
          }
          frame True {
            n127 = call "字符串入队列操作.vi"("字符消息入队列"="退出", "界面切换队列"=w363) -> ()  [unwired: 9 in, 1 out]
            n128 = call "字符串入队列操作.vi"("字符消息入队列"="写退出", "界面切换队列"=w364) -> ()  [unwired: 9 in, 1 out]
          }
        }
        n129 = event-data("Discard?"=TRUE ("放弃？")) -> ()  [unwired: 1 in, 1 out]
      }
    }
  }
  n130 = disable-structure shown="禁用" {
    frame Disabled {
      (unwired) u32 1 ("转换比例")
      (unwired) FALSE ("忽略数值上下限")
      n131 = call "批量读D+10个+16位.vi"() -> ()  [unwired: 8 in, 4 out]
      n132 = call "布尔切换型入队.vi"() -> ()  [unwired: 12 in]
      n133 = call "布尔复位型入队.vi"() -> ()  [unwired: 6 in, 3 out]
      n134 = call "批量读D+5个+32位.vi"() -> ()  [unwired: 8 in, 4 out]
      n135 = call "读D16位.vi"() -> ()  [unwired: 8 in, 4 out]
      n136 = call "写触点.vi"() -> ()  [unwired: 9 in, 3 out]
      n137 = call "写D+32位.vi"() -> ()  [unwired: 8 in, 4 out]
      n138 = call "读D32位.vi"() -> ()  [unwired: 9 in, 3 out]
      n139 = call "读触点-8位.vi"() -> ()  [unwired: 8 in, 4 out]
      n140 = call "界面切换.vi"() -> ()  [unwired: 11 in, 1 out]
      n141 = call "数值输入窗口.vi"() -> ()  [unwired: 13 in, 3 out]
      n142 = call "数值输入窗口.vi"() -> ()  [unwired: 13 in, 3 out]
      n143 = call "数值输入窗口.vi"("输入下限"=0.0, "输入上限"=9999.0, "数据类型"=enum16{"32位", "16位"}."32位") -> ("转换比例"=w370:u32)  [unwired: 9 in, 3 out]
      n144 = call "数值输入窗口.vi"() -> ()  [unwired: 13 in, 3 out]
      n145 = call "数值输入窗口.vi"() -> ()  [unwired: 13 in, 3 out]
      n146 = call "数值输入窗口.vi"() -> ()  [unwired: 13 in, 3 out]
    }
    frame Enabled {
    }
  }
  n147 = disable-structure shown="禁用" {
    frame Disabled {
      n148 = call "读触点-8位.vi"() -> ()  [unwired: 8 in, 4 out]
      n149 = call "写D+32位.vi"() -> ()  [unwired: 8 in, 4 out]
      n150 = call "批量读D+10个+16位.vi"() -> ()  [unwired: 8 in, 4 out]
      n151 = call "写D+16位.vi"() -> ()  [unwired: 7 in, 5 out]
      n152 = call "批量读D+5个+32位.vi"() -> ()  [unwired: 8 in, 4 out]
      n153 = call "字符串入队列操作.vi"() -> ()  [unwired: 11 in, 1 out]
      n154 = call "读D16位.vi"() -> ()  [unwired: 8 in, 4 out]
      n155 = call "读D32位.vi"() -> ()  [unwired: 9 in, 3 out]
      n156 = call "写触点.vi"() -> ()  [unwired: 9 in, 3 out]
      n157 = call "写触点.vi"() -> ()  [unwired: 9 in, 3 out]
    }
    frame Enabled {
    }
  }
  n158 = disable-structure shown="禁用" {
    frame Disabled {
      n159 = for {
        i -> [w372]
        n160 = case shown="9" w372 {
          frame 0, Default {
          }
          frame 1 {
          }
          frame 2 {
          }
          frame 3 {
          }
          frame 4 {
          }
          frame 5 {
          }
          frame 6 {
          }
          frame 7 {
          }
          frame 8 {
          }
          frame 9 {
          }
        }
      }
      n161 = for {
        i -> [w371]
        n162 = case shown="7" w371 {
          frame 0, Default {
          }
          frame 1 {
          }
          frame 2 {
          }
          frame 3 {
          }
          frame 4 {
          }
          frame 5 {
          }
          frame 6 {
          }
          frame 7 {
          }
        }
      }
    }
    frame Enabled {
    }
  }
  n163 = while {
    tunnel: w13 -> [w376]
    tunnel: w12 -> [w375]
    tunnel: w5 -> [w374]
    stop <- TRUE stop-if-true
    n164 = control-ref of="本VI"() -> (w377:refnum<vi>)
    n165 = Release Queue(queue=w374) -> ()  [unwired: 2 in, 3 out]
    n166 = property on="手动界面" class="Bool"("DisabledEnum"=T3."Enabled" ("禁用")) -> ()  [unwired: 2 in, 2 out]
    n167 = invoke class="VI" method="FP.Close"(reference=w377) -> ()  [unwired: 2 in, 3 out]
    "VISA资源名称输出" <- w376
    "错误输出" <- w375
  }
